vi "Set Washer Status.vi"(10 "Washer Data In":T1, 11 "Debug Log":string) -> (2 "Washer Data Out":T1)   [LabVIEW 2011]
uses:
  HCC Data.ctl
  Washer Status Ctrl.ctl
  Globals HCC.vi
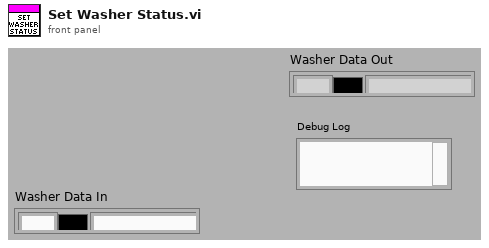
[diagram p1: front panel]
types:
  T1 = typedef "HCC Data.ctl" = cluster{"Station":string, "Color":u32, "Status":T2, "Error Time":string, "Com Err Count":u32, "Debug Log":string}
  T2 = typedef "Washer Status Ctrl.ctl" = enum16{"Running", "Err", "No Com", "No Conf"}
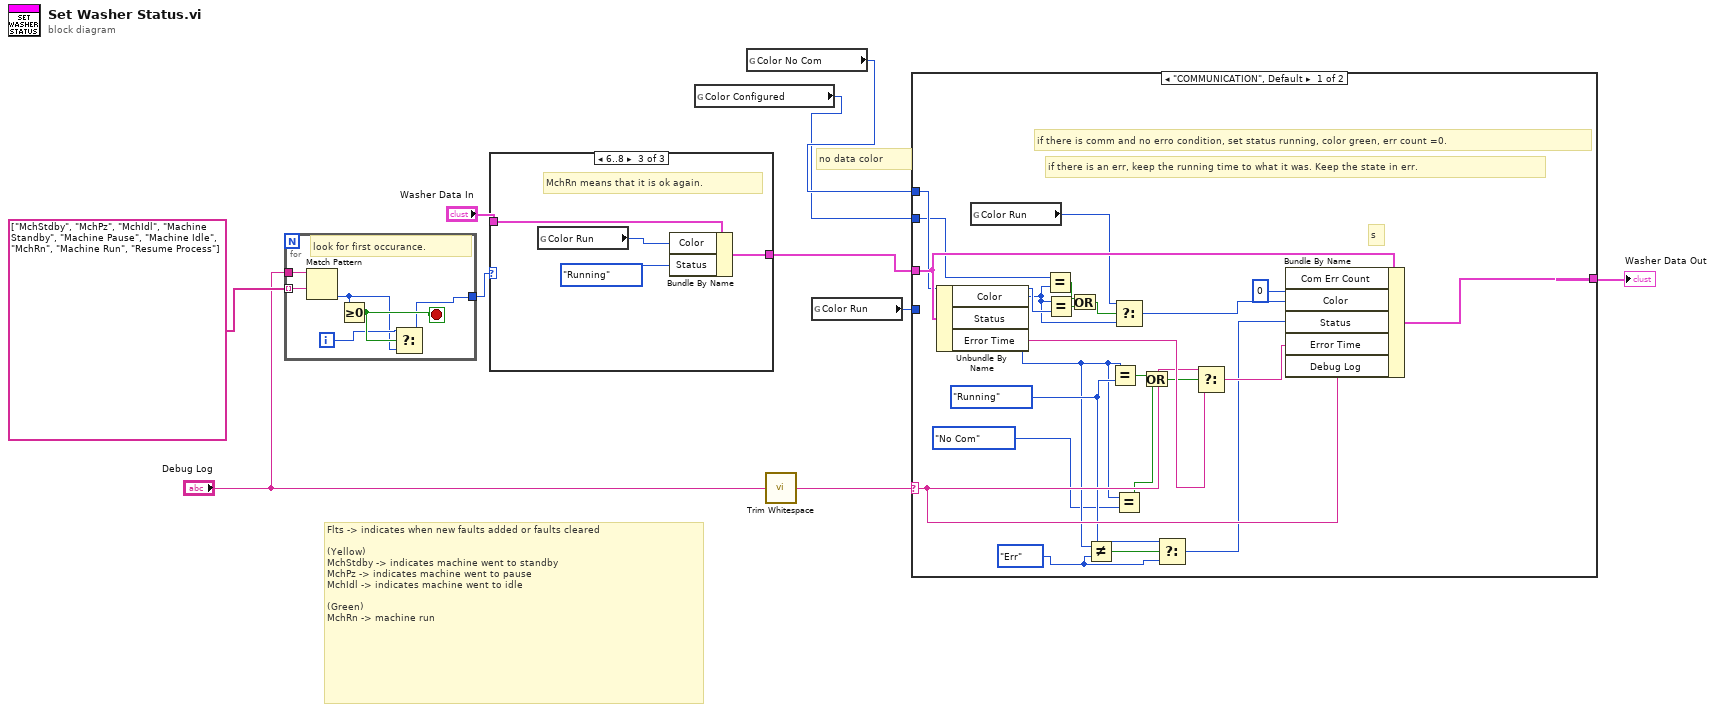
[diagram p0: block diagram]
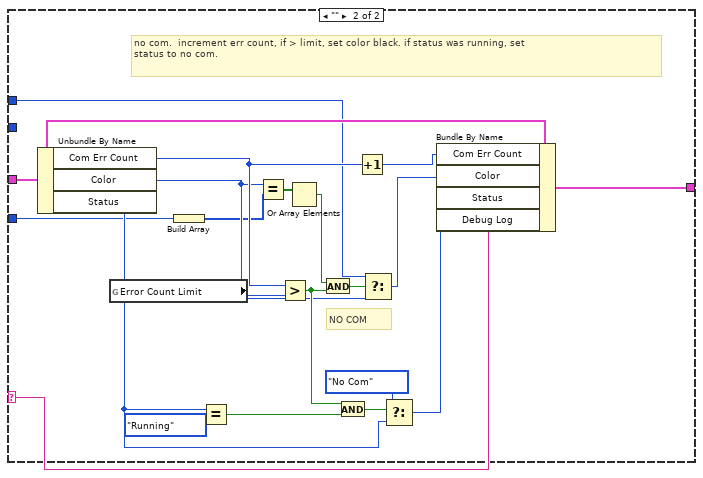
[diagram p2: hidden frame]
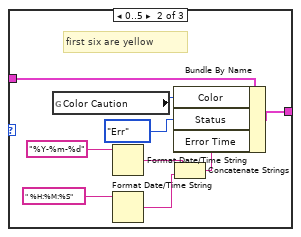
[diagram p4: hidden frame]
diagram:
  # "no data color"
  # "Flts -> indicates when new faults added or faults cleared\n\n(Yellow)\nMchStdby -> indicates machine went to standby\nMchPz -> indicates machine went to pause\nMchIdl -> indicates machine went to idle \n\n(Green)\nMchRn -> machine run"
  n1 = for {
    tunnel: string[] ["MchStdby", "MchPz", "MchIdl", "Machine Standby", "Machine Pause", "Machine Idle", "MchRn", "Machine Run", "Resume Process"] ("operators (none)") -> [w15] mode=indexing
    tunnel: [w12] -> w9
    tunnel: "Debug Log" -> [w16]
    i -> [w13]
    stop <- w14 stop-if-true
    # "look for first occurance."
    n2 = Match Pattern(string=w16, regular expression=w15) -> (offset past match=w11:i32)  [unwired: 1 in, 3 out]
    n3 = Greater Or Equal To 0?(x=w11) -> (x >= 0?=w14:bool)
    n4 = Select(t=w13, s=w14, f=w11) -> (s? t:f=w12:i32)
  }
  n5 = case shown="6..8" w9 {
    tunnel: [w17 w24 w28] -> w3
    tunnel: "Washer Data In" -> [w17 w26 w30]
    frame -1, Default {
      # "Strings not found do nothing."
    }
    frame 0..5 {
      # "first six are yellow"
      n6 = global read "Globals HCC.vi" "Color Caution"() -> (w25:u32)
      n7 = Format Date/Time String(time format string (%c)="%Y-%m-%d") -> (date/time string=w20:string)  [unwired: 2 out]
      n8 = Format Date/Time String(time format string (%c)=" %H:%M:%S") -> (date/time string=w19:string)  [unwired: 2 out]
      n9 = Concatenate Strings(w20, w19) -> (w18:string)
      n10 = Bundle By Name(cluster=w26, "Color"=w25, "Status"=Washer_Status_Ctrl."Err", "Error Time"=w18) -> (w24:T1)
    }
    frame 6..8 {
      # "MchRn means that it is ok again."
      n11 = global read "Globals HCC.vi" "Color Run"() -> (w29:u32)
      n12 = Bundle By Name(cluster=w30, "Color"=w29, "Status"=Washer_Status_Ctrl."Running") -> (w28:T1)
    }
  }
  n13 = global read "Globals HCC.vi" "Color Configured"() -> (w2:u32)
  n14 = global read "Globals HCC.vi" "Color No Com"() -> (w4:u32)
  n15 = call <vilib>:"Trim Whitespace.vi"("string"="Debug Log") -> ("trimmed string"=w5:string)  [unwired: 1 in]
  n16 = global read "Globals HCC.vi" "Color Run"() -> (w1:u32)
  n17 = case shown="\"COMMUNICATION\", Default" w5 {
    selector: w5 -> [w43 w59]
    tunnel: [w53 w73] -> w6
    tunnel: w3 -> [w51 w74]
    tunnel: w4 -> [w50 w67]
    tunnel: w2 -> [w35 _]
    tunnel: w1 -> [_ w57]
    frame "COMMUNICATION", Default {
      w40 = Washer_Status_Ctrl."Err" ("Status")
      w41 = Washer_Status_Ctrl."Running" ("Status")
      # "s"
      # "if there is an err, keep the running time to what it was. Keep the state in err."
      # "if there is comm and no erro condition, set status running, color green, err count =0."
      n18 = Unbundle By Name(w51) -> ("Color"=w36:u32, "Status"=w33:T2, "Error Time"=w44:string)
      n19 = global read "Globals HCC.vi" "Color Run"() -> (w48:u32)
      n20 = Equal?(x=w35, y=w36) -> (x = y?=w37:bool)
      n21 = Equal?(x=w36, y=w50) -> (x = y?=w49:bool)
      n22 = Or(x=w37, y=w49) -> (x .or. y?=w38:bool)
      n23 = Not Equal?(x=w33, y=w40) -> (x != y?=w42:bool)
      n24 = Equal?(x=w33, y=w41) -> (x = y?=w46:bool)
      n25 = Select(t=w48, s=w38, f=w36) -> (s? t:f=w47:u32)
      n26 = Equal?(x=w33, y=Washer_Status_Ctrl."No Com") -> (x = y?=w31:bool)
      n27 = Or(x=w46, y=w31) -> (x .or. y?=w34:bool)
      n28 = Select(t=w41, s=w42, f=w40) -> (s? t:f=w39:T2)
      n29 = Select(t=w43, s=w34, f=w44) -> (s? t:f=w45:string)
      n30 = Bundle By Name(cluster=w51, "Com Err Count"=u32 0 ("Err Count"), "Color"=w47, "Status"=w39, "Error Time"=w45, "Debug Log"=w43) -> (w53:T1)
    }
    frame "" {
      # "no com.  increment err count, if > limit, set color black. if status was running, set\nstatus to no com."
      # "NO COM"
      n31 = Unbundle By Name(w74) -> ("Com Err Count"=w71:u32, "Color"=w55:u32, "Status"=w63:T2)
      n32 = global read "Globals HCC.vi" "Error Count Limit"() -> (w70:u32)
      n33 = Build Array(w57) -> (w54:u32[])
      n34 = Equal?(x=w63, y=Washer_Status_Ctrl."Running") -> (x = y?=w65:bool)
      n35 = Equal?(x=w55, y=w54) -> (x = y?=w56:bool[])
      n36 = Greater?(x=w71, y=w70) -> (0:w66:bool)
      n37 = Or Array Elements(Boolean array=w56) -> (logical OR=w58:bool)
      n38 = And(x=w58, y=w66) -> (x .and. y?=w69:bool)
      n39 = And(x=w66, y=w65) -> (x .and. y?=w64:bool)
      n40 = Increment(x=w71) -> (x+1=w72:u32)
      n41 = Select(t=w67, s=w69, f=w55) -> (s? t:f=w68:u32)
      n42 = Select(t=Washer_Status_Ctrl."No Com" ("Status"), s=w64, f=w63) -> (s? t:f=w62:T2)
      n43 = Bundle By Name(cluster=w74, "Com Err Count"=w72, "Color"=w68, "Status"=w62, "Debug Log"=w59) -> (w73:T1)
    }
  }
  "Washer Data Out" <- w6
